vi "Initialize (NVMEM Area).vi"(0 "NVMEM areas":refnum<k21>, 7 "reservation access (Read/Write)":i32(ring)=3 items=["None"=0, "Read Only"=1, "Read/Write"=3], 9 "reservation group":string, 11 "error in (no error)":errorcluster, 12 "connect timeout (60 sec)":dbl=60.0) -> (4 "SLSC Local out":refnum<class "SLSC Local.lvclass">, 15 "error out":errorcluster)   [LabVIEW 2015, in "SLSC Local.lvclass"]
uses:
  SLSC Local.lvclass
  SLSC Local.lvclass/SLSC Local.ctl
  <vilib>/SLSC/Initialize Session with NVMEM Areas.vi
  <vilib>/SLSC/SLSC.lvlib
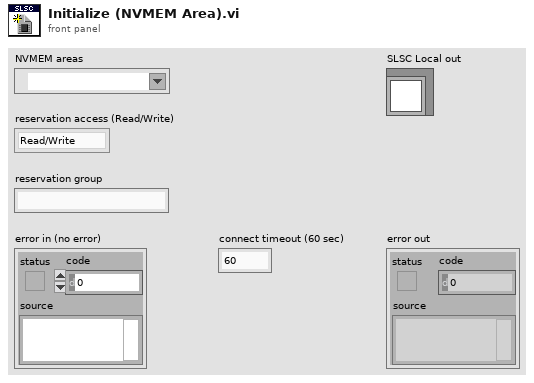
[diagram p1: front panel]
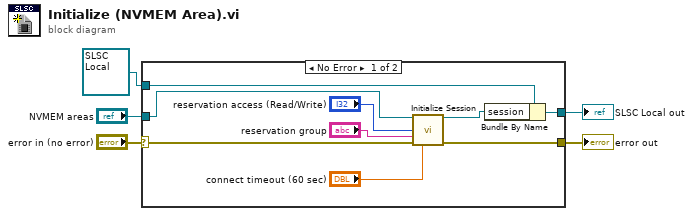
[diagram p0: block diagram]
diagram:
  n1 = case shown="No Error" "error in (no error)" {
    selector: "error in (no error)" -> [w12 w16]
    tunnel: [w11 w16] -> w4
    tunnel: [w13 w15] -> w2
    tunnel: refnum<class "SLSC Local.lvclass"> refnum ("SLSC Local in") -> [w14 w15]
    tunnel: "NVMEM areas" -> [w6 _]
    frame No Error {
      n2 = call-poly <vilib>:"Initialize Session.vi"("NVMEM areas"=w6, "reservation access (Read/Write)"="reservation access (Read/Write)", "reservation group"="reservation group", "error in (no error)"=w12, "connect timeout (60 sec)"="connect timeout (60 sec)") -> ("session out"=w10:refnum<k21>, "error out"=w11:errorcluster)  [unwired: 9 in]
      n3 = Bundle By Name(cluster=w14, "session"=w10) -> (w13:refnum<class "SLSC Local.lvclass">)
    }
    frame Error {
    }
  }
  "error out" <- w4
  "SLSC Local out" <- w2
